vi "Get Multiple Attributes from Variant.vi"(8 "error in":errorcluster, 10 "Keys":string[](array[string]), 11 "Variant in":variant) -> (0 "error out":errorcluster, 2 "Values":variant[](array[variant]))   [LabVIEW 2020, in "hse-misc.lvlib"]
doc: "____\nHAMPEL SOFTWARE ENGINEERING v3.8.0 (2023-12-18 14:41)"
uses:
  hse-misc.lvlib
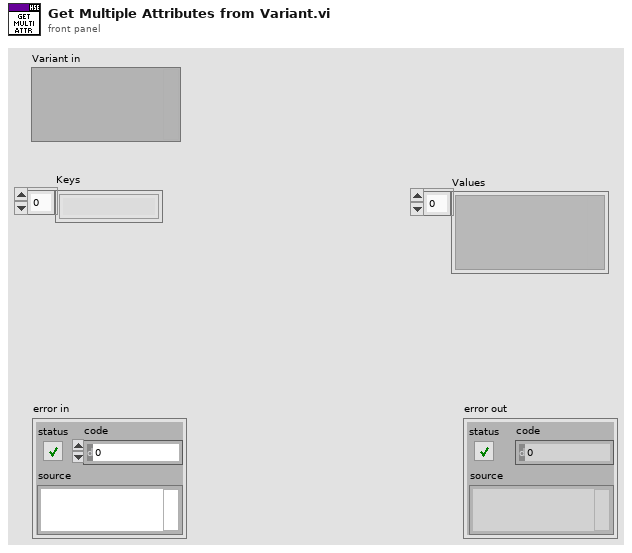
[diagram p1: front panel]
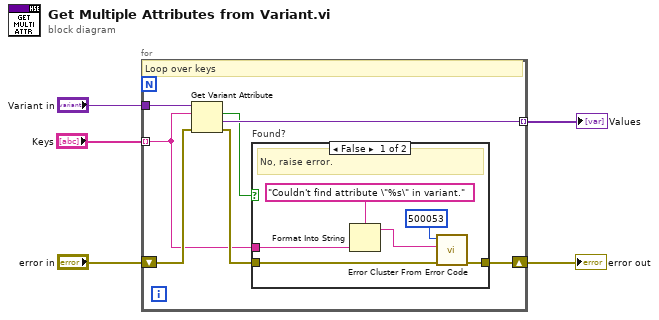
[diagram p0: block diagram]
diagram:
  n1 = for {
    shift-right: [w7] -> w2
    shift-left: "error in" -> [w12]
    tunnel: "Keys" -> [w6] mode=indexing
    tunnel: [w11] -> w1 mode=indexing
    tunnel: "Variant in" -> [w10]
    # "Loop over keys"
    n2 = Get Variant Attribute(Variant=w10, name=w6, error in=w12) -> (found=w9:bool, value=w11:variant, error out=w8:errorcluster)  [unwired: 1 in, 1 out]
    n3 = case "Found?" shown="False" w9 {
      tunnel: w8 -> [w18 w19]
      tunnel: [w17 w19] -> w7
      tunnel: w6 -> [w13 _]
      frame False {
        # "No, raise error."
        n4 = Format Into String(format string="Couldn't find attribute \"%s\" in variant.", w13) -> (resulting string=w14:string)  [unwired: 2 in, 1 out]
        n5 = call <vilib>:"Error Cluster From Error Code.vi"("error in (no error)"=w18, "error message (\"\")"=w14, "error code (0)"=500053) -> ("error out"=w17:errorcluster)  [unwired: 6 in]
      }
      frame True {
        # "Yes"
      }
    }
  }
  "error out" <- w2
  "Values" <- w1
